vi "LRC checker.vi"(11 "Data In":u8[](array[numeric])) -> (2 "Valid?":bool, 3 "Function Data Out":u8[](array[numeric]))   [LabVIEW 2012, in "ASCII Data Unit.lvclass"]
doc: "this is where the magic happens."
uses:
  ASCII Data Unit.lvclass
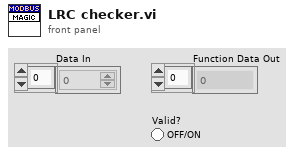
[diagram p1: front panel]
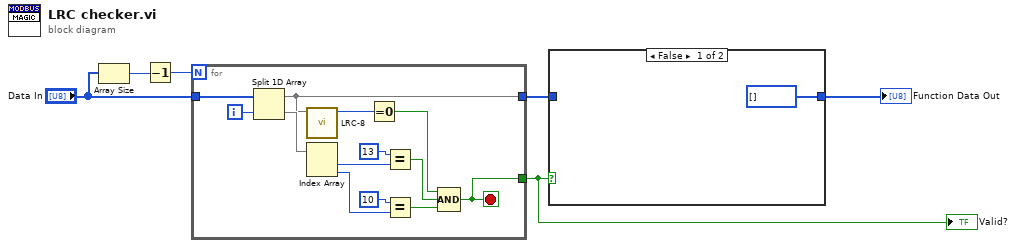
[diagram p0: block diagram]
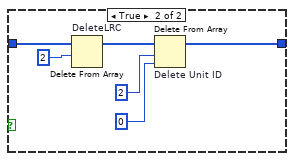
[diagram p2: hidden frame]
diagram:
  n1 = Array Size(array="Data In") -> (size(s)=w5:i32)
  n2 = Decrement(x=w5) -> (x-1=w4:i32)
  n3 = for {
    N: w4 -> [_]
    tunnel: "Data In" -> [w15]
    tunnel: [w8] -> w3
    tunnel: [w7] -> w2
    i -> [w14]
    stop <- w7 stop-if-true
    n4 = Split 1D Array(array=w15, index=w14) -> (first subarray=w8:u8[], second subarray=w13:u8[])
    n5 = call "LRC-8.vi"("data"=w8) -> ("LRC-8"=w12:u8)  [unwired: 10 in]
    n6 = Index Array(array=w13) -> (element #1=w19:u8, element #2=w16:u8)  [unwired: 2 in]
    n7 = Equal To 0?(x=w12) -> (x = 0?=w11:bool)
    n8 = Equal?(x=u8 13, y=w19) -> (x = y?=w10:bool)
    n9 = Equal?(x=u8 10, y=w16) -> (x = y?=w9:bool)
    n10 = Compound Arithmetic op=AND(w11, w10, w9) -> (w7:bool)
  }
  "Valid?" <- w2
  n11 = case shown="False" w2 {
    tunnel: w3 -> [_ w22]
    tunnel: [u8[] [] w21] -> w1
    frame False {
    }
    frame True {
      n12 = Delete From Array "DeleteLRC"(array=w22, length=2) -> (array with subset deleted=w24:u8[])  [unwired: 1 in, 1 out]
      n13 = Delete From Array "Delete Unit ID"(array=w24, length=2, index=0) -> (array with subset deleted=w21:u8[])  [unwired: 1 out]
    }
  }
  "Function Data Out" <- w1
